vi "LKIF_SetZero.vi"(7 "OutNo (OUT1)":T1 items=["OUT1", "OUT2", "OUT1+OUT2"], 8 "error in (no error)":errorcluster {"code" format="%x"}, 11 "IsOn":bool) -> (0 "error out":errorcluster {"code" format="%x"})   [LabVIEW 2024, in "Keyence LK-G3000.lvlib"]
uses:
  Keyence LK-G3000.lvlib
  enums/LKIF_OUTNO.ctl
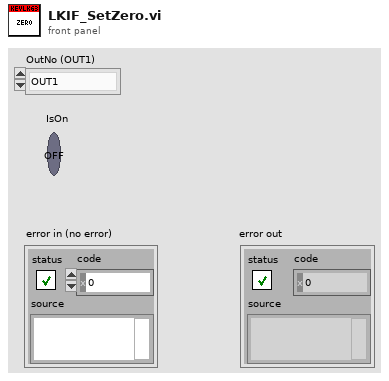
[diagram p1: front panel]
types:
  T1 = typedef "Keyence LK-G3000.lvlib/LKIF_OUTNO.ctl" = i32
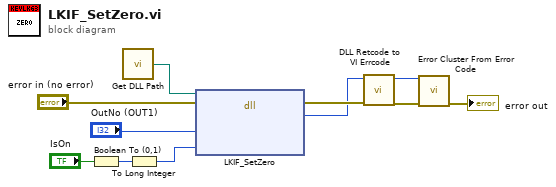
[diagram p0: block diagram]
diagram:
  n1 = Boolean To (0,1)(Boolean="IsOn") -> (0, 1=w7:i16)
  n2 = call "Get DLL Path.vi"() -> ("DLL Path"=w2:path)  [unwired: 1 in]
  n3 = To Long Integer(number=w7) -> (32bit integer=w4:i32)
  n4 = dll-call lib="C:/Program Files/National Instruments/LabVIEW 2011/instr.lib/Keyence LK-G3000/LkIF.dll" fn="LKIF_SetZero"(path in=w2, error in="error in (no error)", "OutNo"="OutNo (OUT1)", "IsOn"=w4) -> (error out=w6:errorcluster, "RC"=w3:i32)  [unwired: 3 in, 1 out]
  n5 = call "DLL Retcode to VI Errcode.vi"("error in (no error)"=w6, "DLL Retcode"=w3) -> ("error out"=w11:errorcluster, "VI Errcode"=w10:i32)  [unwired: 8 in]
  n6 = call <vilib>:"Error Cluster From Error Code.vi"("error in (no error)"=w11, "error code (0)"=w10) -> ("error out"=→"error out":errorcluster)  [unwired: 7 in]
